vi "sub vi - Read Analog All v8.vi"(0 "Task0":dbl, 5 "Task1":dbl, 7 "Task2":dbl, 9 "Samples":dbl) -> (2 "Analog loop time":dbl, 3 "array GRAPH":dynamicdata[](array[waveform]), 4 "LAB01":T2, 6 "LAB02":T3, 8 "LAB03":T4, 10 "LAB04":T5, 13 "deg C":dbl, 14 "array ERROR":errorcluster[](array[cluster]), 15 "LAB05":T6)   [LabVIEW 2013]
uses:
  <vilib>/addons/Electrical Power/Basic/Measurement/Power (1 Channel).vi
  <vilib>/addons/Electrical Power/Basic/Measurement/RMS (N Channels).vi
  <vilib>/addons/Electrical Power/Basic/Measurement/RMS (1 Channel).vi
  <vilib>/addons/Electrical Power/Basic/NI_EP_Basic.lvlib
panel:
  in  "Tab Control":T1(tab)
  out "LAB01-2 (PF)":dbl
  out "LAB01-1 (PF)":dbl
  out "LAB01-2 (V)":dbl
  out "LAB01-2 (A)":dbl
  out "LAB01-1 (V)":dbl
  out "LAB01-1 (A)":dbl
  out "LAB01-2 (GRAPH)":dynamicdata(graph)
  out "LAB01-1 (GRAPH)":dynamicdata(graph)
  out "LAB02-2 (PF)":dbl
  out "LAB02-1 (PF)":dbl
  out "LAB02-2 (V)":dbl
  out "LAB02-2 (A)":dbl
  out "LAB02-1 (V)":dbl
  out "LAB02-1 (A)":dbl
  out "LAB02-2 (GRAPH)":dynamicdata(graph)
  out "LAB02-1 (GRAPH)":dynamicdata(graph)
  out "LAB03-2 (PF)":dbl
  out "LAB03-1 (PF)":dbl
  out "LAB03-2 (V)":dbl
  out "LAB03-2 (A)":dbl
  out "LAB03-1 (V)":dbl
  out "LAB03-1 (A)":dbl
  out "LAB03-2 (GRAPH)":dynamicdata(graph)
  out "LAB03-1 (GRAPH)":dynamicdata(graph)
  out "LAB04-2 (PF)":dbl
  out "LAB04-1 (PF)":dbl
  out "LAB04-2 (V)":dbl
  out "LAB04-2 (A)":dbl
  out "LAB04-1 (V)":dbl
  out "LAB04-1 (A)":dbl
  out "LAB04-1 (GRAPH)":dynamicdata(graph)
  out "LAB04-2 (GRAPH)":dynamicdata(graph)
  out "LAB05-2 (PF)":dbl
  out "LAB05-1 (PF)":dbl
  out "LAB05-2 (V)":dbl
  out "LAB05-2 (A)":dbl
  out "LAB05-1 (V)":dbl
  out "LAB05-1 (A)":dbl
  out "LAB05-1 (GRAPH)":dynamicdata(graph)
  out "LAB05-2 (GRAPH)":dynamicdata(graph)
  out "A1 error":errorcluster
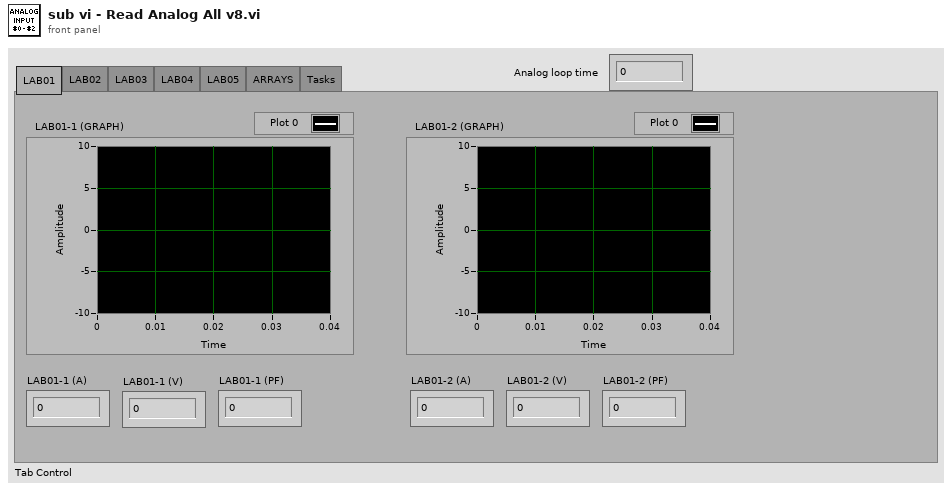
[diagram p1: front panel]
types:
  T1 = enum32{"LAB01", "LAB02", "LAB03", "LAB04", "LAB05", "ARRAYS", "Tasks"}
  T2 = cluster{"LAB01-1 (A)":dbl, "LAB01-1 (V)":dbl, "LAB01-1 (PF)":dbl, "LAB01-2 (A)":dbl, "LAB01-2 (V)":dbl, "LAB01-2 (PF)":dbl}
  T3 = cluster{"LAB02-1 (A)":dbl, "LAB02-1 (V)":dbl, "LAB02-1 (PF)":dbl, "LAB02-2 (A)":dbl, "LAB02-2 (V)":dbl, "LAB02-2 (PF)":dbl}
  T4 = cluster{"LAB03-1 (A)":dbl, "LAB03-1 (V)":dbl, "LAB03-1 (PF)":dbl, "LAB03-2 (A)":dbl, "LAB03-2 (V)":dbl, "LAB03-2 (PF)":dbl}
  T5 = cluster{"LAB04-1 (A)":dbl, "LAB04-1 (V)":dbl, "LAB04-1 (PF)":dbl, "LAB04-2 (A)":dbl, "LAB04-2 (V)":dbl, "LAB04-2 (PF)":dbl}
  T6 = cluster{"LAB05-1 (A)":dbl, "LAB05-1 (V)":dbl, "LAB05-1 (PF)":dbl, "LAB05-2 (A)":dbl, "LAB05-2 (V)":dbl, "LAB05-2 (PF)":dbl}
  T7 = typedef "NI_EP_Basic.lvlib/basic_Power Value.ctl" = cluster{"active power [W]":dbl, "apparent power [VA]":dbl, "reactive power [VAR]":dbl, "power factor":dbl}
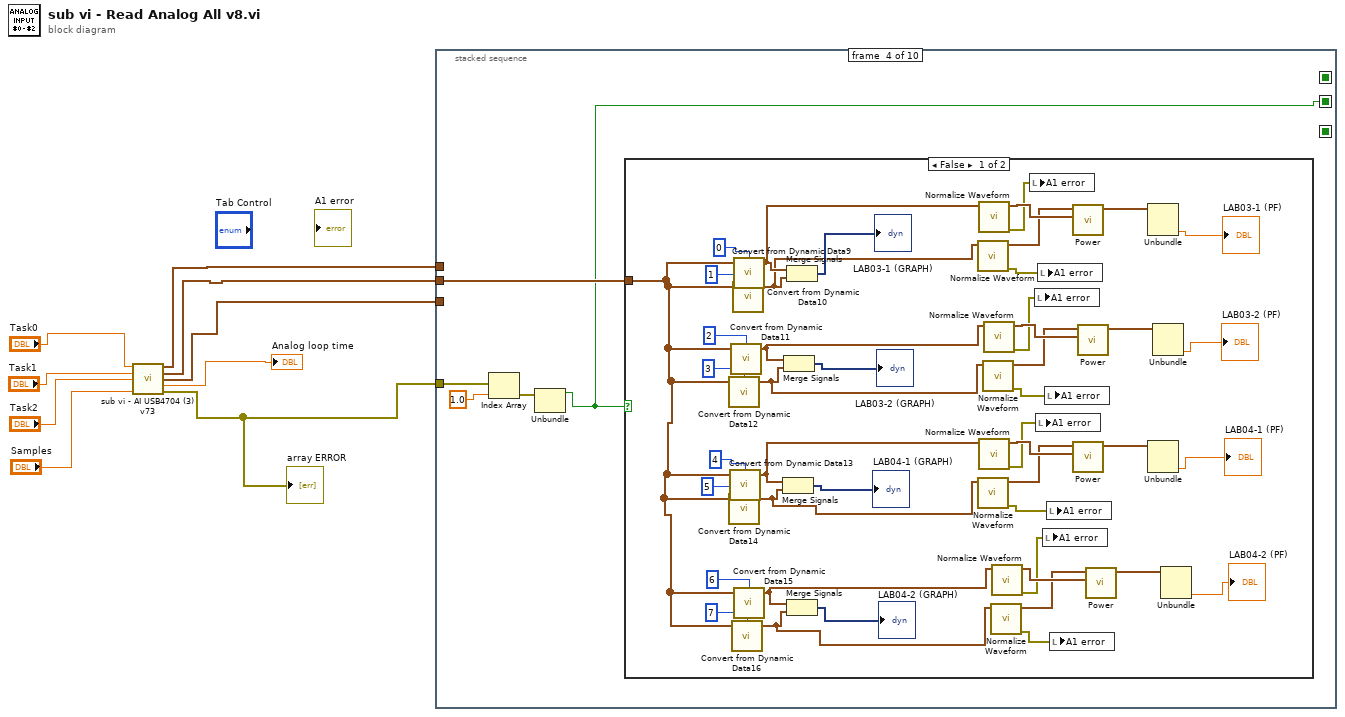
[diagram p0: block diagram]
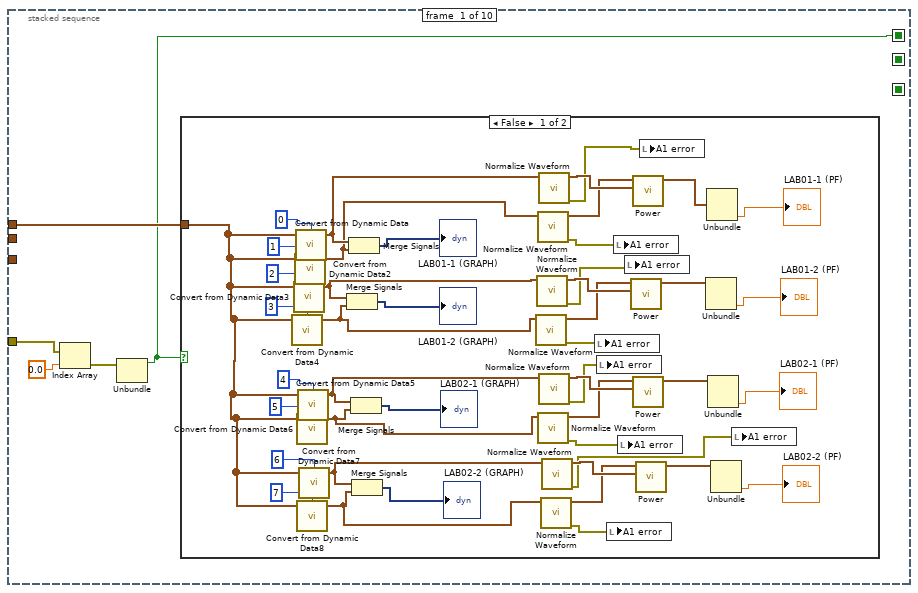
[diagram p2: hidden frame]
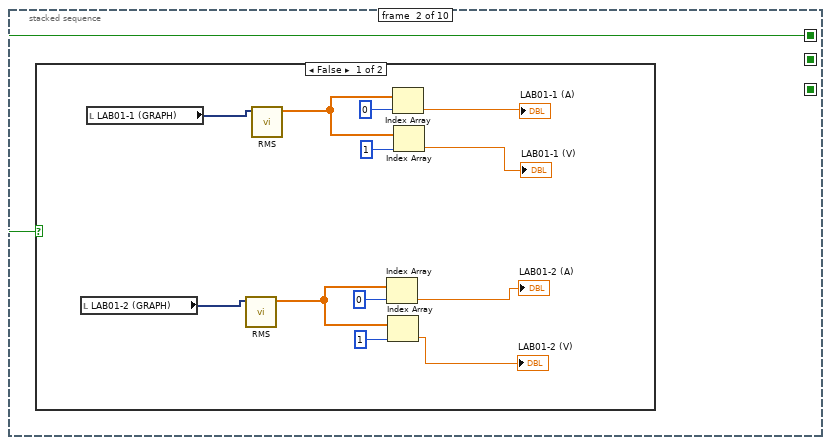
[diagram p4: hidden frame]
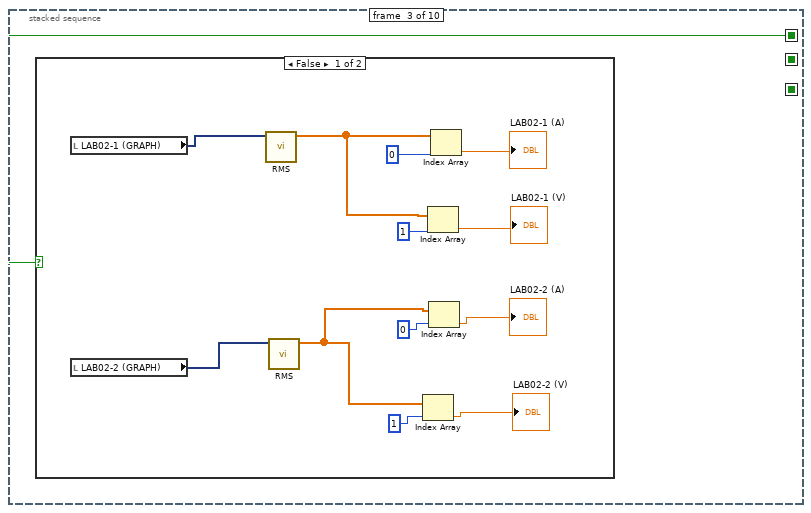
[diagram p6: hidden frame]
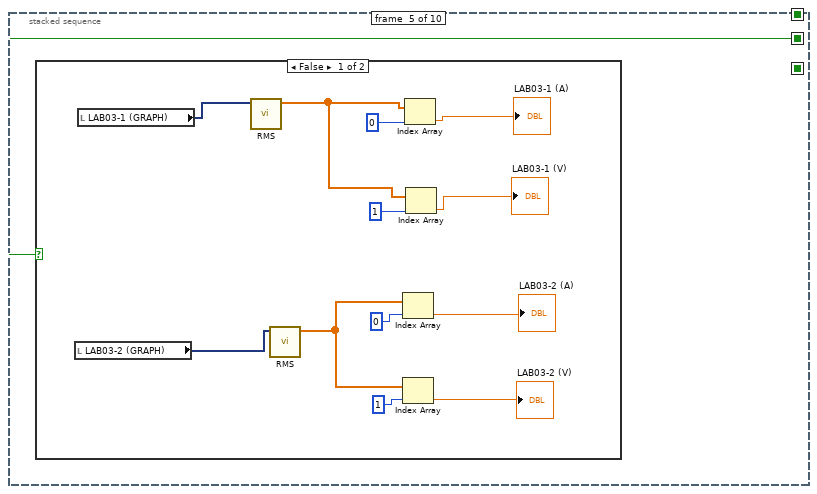
[diagram p9: hidden frame]
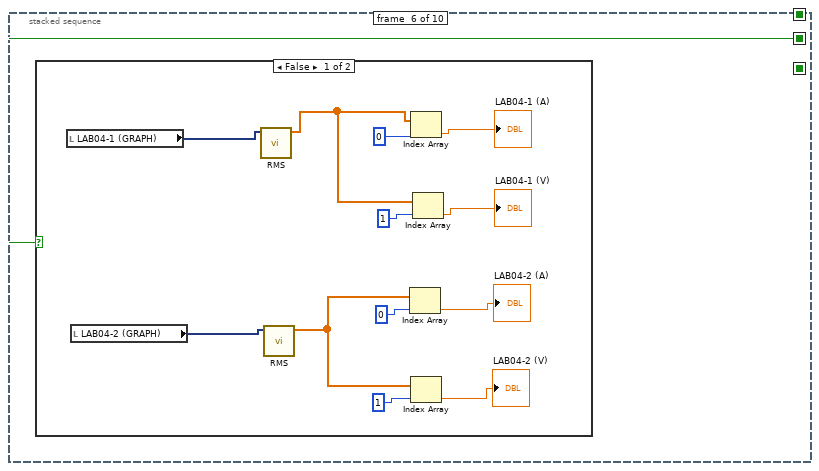
[diagram p11: hidden frame]
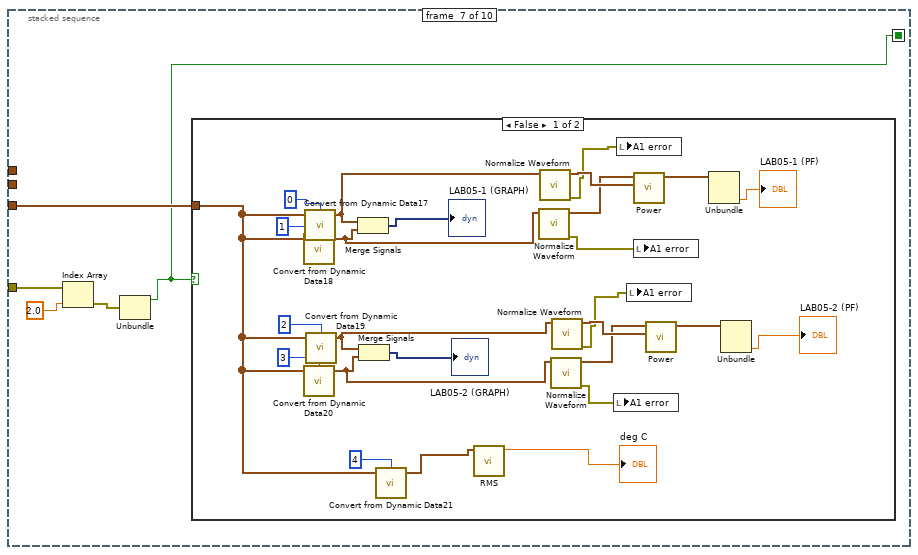
[diagram p13: hidden frame]
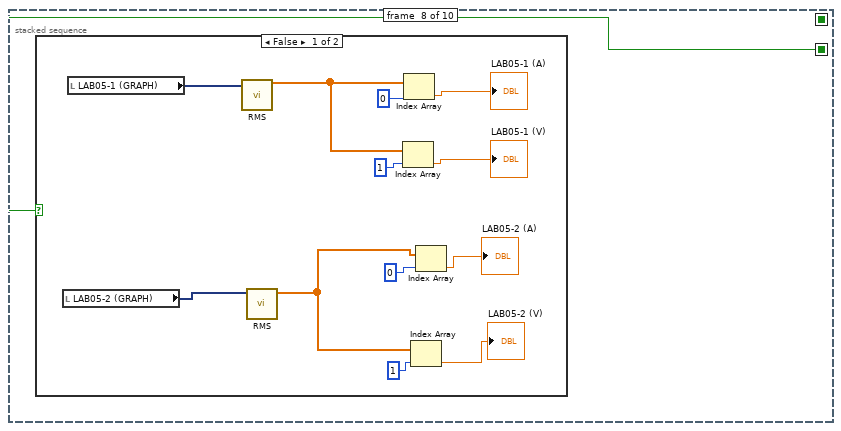
[diagram p15: hidden frame]
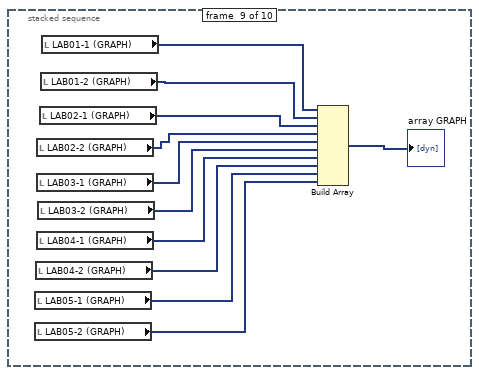
[diagram p17: hidden frame]
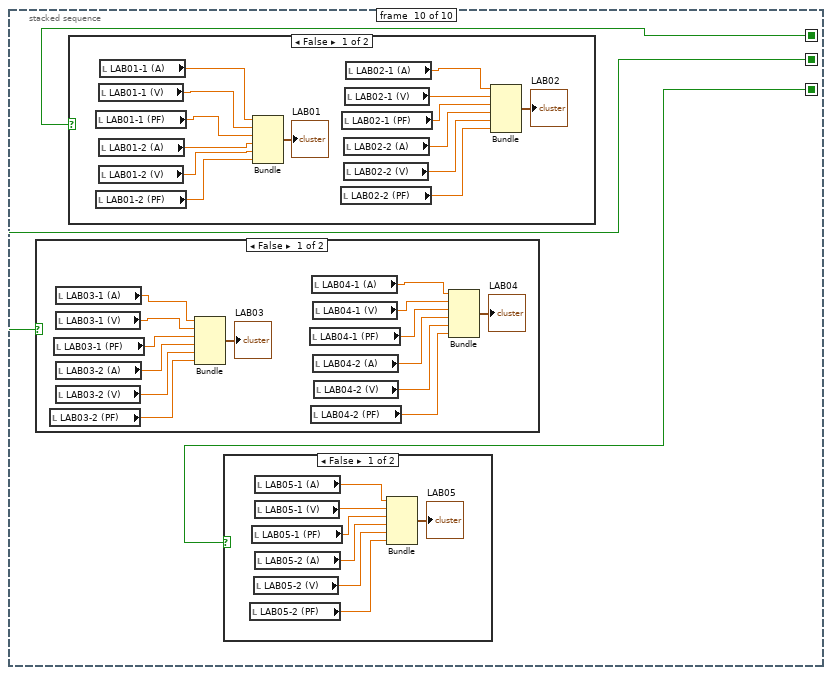
[diagram p18: hidden frame]
diagram:
  n1 = call "sub vi - AI USB4704 (3) v73.vi"("Task0"="Task0", "Task1"="Task1", "Task2"="Task2", "SAMPLES"="Samples") -> ("data 0"=w9:waveform(dbl)[], "data 1"=w8:waveform(dbl)[], "data 2"=w7:waveform(dbl)[], "loop time"=→"Analog loop time":dbl, "error array"=w5:errorcluster[])  [unwired: 7 in]
  "array ERROR" <- w5
  n2 = stacked-sequence {
    seq-local: [w10 _ _ _ _ _ _ _ _ _] -> [_ w60 w73 _ _ _ _ _ _ w219]
    seq-local: [_ _ _ w86 _ _ _ _ _ _] -> [_ _ _ _ w136 w149 _ _ _ w218]
    seq-local: [_ _ _ _ _ _ w162 _ _ _] -> [_ _ _ _ _ _ _ w193 _ w217]
    tunnel: w9 -> [w14 _ _ _ _ _ _ _ _ _]
    tunnel: w8 -> [_ _ _ w90 _ _ _ _ _ _]
    tunnel: w7 -> [_ _ _ _ _ _ w166 _ _ _]
    tunnel: w5 -> [w13 _ _ w89 _ _ w165 _ _ _]
    frame #0 {
      n3 = Index Array(array=w13, index=0.0) -> (element=w11:errorcluster)
      n4 = Unbundle(w11) -> ("status"=w10:bool)  [unwired: 2 out]
      n5 = case shown="False" w10 {
        tunnel: w14 -> [w49 _]
        frame False {
          n6 = call "Convert from Dynamic Data4"("Dynamic Data Type"=w49, "Channel"=3) -> ("Waveform"=w35:waveform(dbl))  [unwired: 2 in]
          n7 = call "Convert from Dynamic Data3"("Dynamic Data Type"=w49, "Channel"=2) -> ("Waveform"=w36:waveform(dbl))  [unwired: 2 in]
          n8 = call "Convert from Dynamic Data2"("Dynamic Data Type"=w49, "Channel"=1) -> ("Waveform"=w45:waveform(dbl))  [unwired: 2 in]
          n9 = call "Convert from Dynamic Data"("Dynamic Data Type"=w49, "Channel"=0) -> ("Waveform"=w46:waveform(dbl))  [unwired: 2 in]
          n10 = call "Convert from Dynamic Data6"("Dynamic Data Type"=w49, "Channel"=5) -> ("Waveform"=w30:waveform(dbl))  [unwired: 2 in]
          n11 = call "Convert from Dynamic Data8"("Dynamic Data Type"=w49, "Channel"=7) -> ("Waveform"=w24:waveform(dbl))  [unwired: 2 in]
          n12 = call "Convert from Dynamic Data5"("Dynamic Data Type"=w49, "Channel"=4) -> ("Waveform"=w31:waveform(dbl))  [unwired: 2 in]
          n13 = call "Convert from Dynamic Data7"("Dynamic Data Type"=w49, "Channel"=6) -> ("Waveform"=w25:waveform(dbl))  [unwired: 2 in]
          n14 = Merge Signals(w36, w35) -> (→"LAB01-2 (GRAPH)":dynamicdata)
          n15 = Merge Signals(w46, w45) -> (→"LAB01-1 (GRAPH)":dynamicdata)
          n16 = Merge Signals(w31, w30) -> (→"LAB02-1 (GRAPH)":dynamicdata)
          n17 = Merge Signals(w25, w24) -> (→"LAB02-2 (GRAPH)":dynamicdata)
          n18 = call <vilib>:"Normalize Waveform.vi"("waveform in"=w35) -> ("error out"=w19:errorcluster, "normalized waveform"=w39:waveform(dbl))  [unwired: 7 in, 2 out]
          n19 = call <vilib>:"Normalize Waveform.vi"("waveform in"=w36) -> ("error out"=w20:errorcluster, "normalized waveform"=w40:waveform(dbl))  [unwired: 7 in, 2 out]
          n20 = call <vilib>:"Normalize Waveform.vi"("waveform in"=w45) -> ("error out"=w21:errorcluster, "normalized waveform"=w43:waveform(dbl))  [unwired: 7 in, 2 out]
          n21 = call <vilib>:"Normalize Waveform.vi"("waveform in"=w30) -> ("error out"=w17:errorcluster, "normalized waveform"=w33:waveform(dbl))  [unwired: 7 in, 2 out]
          n22 = call <vilib>:"Normalize Waveform.vi"("waveform in"=w46) -> ("error out"=w22:errorcluster, "normalized waveform"=w44:waveform(dbl))  [unwired: 7 in, 2 out]
          n23 = call <vilib>:"Normalize Waveform.vi"("waveform in"=w31) -> ("error out"=w18:errorcluster, "normalized waveform"=w34:waveform(dbl))  [unwired: 7 in, 2 out]
          n24 = call <vilib>:"Normalize Waveform.vi"("waveform in"=w24) -> ("error out"=w15:errorcluster, "normalized waveform"=w27:waveform(dbl))  [unwired: 7 in, 2 out]
          n25 = call <vilib>:"Normalize Waveform.vi"("waveform in"=w25) -> ("error out"=w16:errorcluster, "normalized waveform"=w28:waveform(dbl))  [unwired: 7 in, 2 out]
          n26 = local write "A1 error"(w19) -> ()
          n27 = local write "A1 error"(w18) -> ()
          n28 = local write "A1 error"(w15) -> ()
          n29 = local write "A1 error"(w21) -> ()
          n30 = local write "A1 error"(w17) -> ()
          n31 = local write "A1 error"(w20) -> ()
          n32 = call-poly <vilib>:"Power.vi"("current waveform"=w40, "voltage waveform"=w39) -> ("power value"=w38:T7)  [unwired: 8 in, 1 out]
          n33 = call-poly <vilib>:"Power.vi"("current waveform"=w44, "voltage waveform"=w43) -> ("power value"=w42:T7)  [unwired: 8 in, 1 out]
          n34 = call-poly <vilib>:"Power.vi"("current waveform"=w34, "voltage waveform"=w33) -> ("power value"=w32:T7)  [unwired: 8 in, 1 out]
          n35 = call-poly <vilib>:"Power.vi"("current waveform"=w28, "voltage waveform"=w27) -> ("power value"=w26:T7)  [unwired: 8 in, 1 out]
          n36 = local write "A1 error"(w22) -> ()
          n37 = Unbundle(w38) -> ("power factor"=→"LAB01-2 (PF)":dbl)  [unwired: 3 out]
          n38 = Unbundle(w42) -> ("power factor"=→"LAB01-1 (PF)":dbl)  [unwired: 3 out]
          n39 = Unbundle(w32) -> ("power factor"=→"LAB02-1 (PF)":dbl)  [unwired: 3 out]
          n40 = Unbundle(w26) -> ("power factor"=→"LAB02-2 (PF)":dbl)  [unwired: 3 out]
          n41 = local write "A1 error"(w16) -> ()
        }
        frame True {
        }
      }
    }
    frame #1 {
      n42 = case shown="False" w60 {
        frame False {
          n43 = local read "LAB01-2 (GRAPH)"() -> (w69:dynamicdata)
          n44 = local read "LAB01-1 (GRAPH)"() -> (w63:dynamicdata)
          n45 = call-poly <vilib>:"RMS.vi"("waveforms"=w69) -> ("RMS values"=w68:dbl[])  [unwired: 9 in, 1 out]
          n46 = call-poly <vilib>:"RMS.vi"("waveforms"=w63) -> ("RMS values"=w72:dbl[])  [unwired: 9 in, 1 out]
          n47 = Index Array(array=w68, index=0) -> (element=→"LAB01-2 (A)":dbl)
          n48 = Index Array(array=w68, index=1) -> (element=→"LAB01-2 (V)":dbl)
          n49 = Index Array(array=w72, index=0) -> (element=→"LAB01-1 (A)":dbl)
          n50 = Index Array(array=w72, index=1) -> (element=→"LAB01-1 (V)":dbl)
        }
        frame True {
        }
      }
    }
    frame #2 {
      n51 = case shown="False" w73 {
        frame False {
          n52 = local read "LAB02-1 (GRAPH)"() -> (w81:dynamicdata)
          n53 = local read "LAB02-2 (GRAPH)"() -> (w77:dynamicdata)
          n54 = call-poly <vilib>:"RMS.vi"("waveforms"=w81) -> ("RMS values"=w80:dbl[])  [unwired: 9 in, 1 out]
          n55 = call-poly <vilib>:"RMS.vi"("waveforms"=w77) -> ("RMS values"=w76:dbl[])  [unwired: 9 in, 1 out]
          n56 = Index Array(array=w76, index=1) -> (element=→"LAB02-2 (V)":dbl)
          n57 = Index Array(array=w80, index=1) -> (element=→"LAB02-1 (V)":dbl)
          n58 = Index Array(array=w76, index=0) -> (element=→"LAB02-2 (A)":dbl)
          n59 = Index Array(array=w80, index=0) -> (element=→"LAB02-1 (A)":dbl)
        }
        frame True {
        }
      }
    }
    frame #3 {
      n60 = Index Array(array=w89, index=1.0) -> (element=w87:errorcluster)
      n61 = Unbundle(w87) -> ("status"=w86:bool)  [unwired: 2 out]
      n62 = case shown="False" w86 {
        tunnel: w90 -> [w123 _]
        frame False {
          n63 = call "Convert from Dynamic Data12"("Dynamic Data Type"=w123, "Channel"=3) -> ("Waveform"=w112:waveform(dbl))  [unwired: 2 in]
          n64 = call "Convert from Dynamic Data14"("Dynamic Data Type"=w123, "Channel"=5) -> ("Waveform"=w106:waveform(dbl))  [unwired: 2 in]
          n65 = call "Convert from Dynamic Data13"("Dynamic Data Type"=w123, "Channel"=4) -> ("Waveform"=w107:waveform(dbl))  [unwired: 2 in]
          n66 = call "Convert from Dynamic Data11"("Dynamic Data Type"=w123, "Channel"=2) -> ("Waveform"=w113:waveform(dbl))  [unwired: 2 in]
          n67 = call "Convert from Dynamic Data16"("Dynamic Data Type"=w123, "Channel"=7) -> ("Waveform"=w100:waveform(dbl))  [unwired: 2 in]
          n68 = call "Convert from Dynamic Data10"("Dynamic Data Type"=w123, "Channel"=1) -> ("Waveform"=w118:waveform(dbl))  [unwired: 2 in]
          n69 = call "Convert from Dynamic Data9"("Dynamic Data Type"=w123, "Channel"=0) -> ("Waveform"=w119:waveform(dbl))  [unwired: 2 in]
          n70 = call "Convert from Dynamic Data15"("Dynamic Data Type"=w123, "Channel"=6) -> ("Waveform"=w101:waveform(dbl))  [unwired: 2 in]
          n71 = Merge Signals(w107, w106) -> (→"LAB04-1 (GRAPH)":dynamicdata)
          n72 = Merge Signals(w113, w112) -> (→"LAB03-2 (GRAPH)":dynamicdata)
          n73 = Merge Signals(w119, w118) -> (→"LAB03-1 (GRAPH)":dynamicdata)
          n74 = Merge Signals(w101, w100) -> (→"LAB04-2 (GRAPH)":dynamicdata)
          n75 = call <vilib>:"Normalize Waveform.vi"("waveform in"=w118) -> ("error out"=w97:errorcluster, "normalized waveform"=w121:waveform(dbl))  [unwired: 7 in, 2 out]
          n76 = call <vilib>:"Normalize Waveform.vi"("waveform in"=w106) -> ("error out"=w93:errorcluster, "normalized waveform"=w109:waveform(dbl))  [unwired: 7 in, 2 out]
          n77 = call <vilib>:"Normalize Waveform.vi"("waveform in"=w119) -> ("error out"=w98:errorcluster, "normalized waveform"=w122:waveform(dbl))  [unwired: 7 in, 2 out]
          n78 = call <vilib>:"Normalize Waveform.vi"("waveform in"=w107) -> ("error out"=w94:errorcluster, "normalized waveform"=w110:waveform(dbl))  [unwired: 7 in, 2 out]
          n79 = call <vilib>:"Normalize Waveform.vi"("waveform in"=w112) -> ("error out"=w95:errorcluster, "normalized waveform"=w115:waveform(dbl))  [unwired: 7 in, 2 out]
          n80 = call <vilib>:"Normalize Waveform.vi"("waveform in"=w113) -> ("error out"=w96:errorcluster, "normalized waveform"=w116:waveform(dbl))  [unwired: 7 in, 2 out]
          n81 = call <vilib>:"Normalize Waveform.vi"("waveform in"=w100) -> ("error out"=w91:errorcluster, "normalized waveform"=w103:waveform(dbl))  [unwired: 7 in, 2 out]
          n82 = call <vilib>:"Normalize Waveform.vi"("waveform in"=w101) -> ("error out"=w92:errorcluster, "normalized waveform"=w104:waveform(dbl))  [unwired: 7 in, 2 out]
          n83 = local write "A1 error"(w98) -> ()
          n84 = local write "A1 error"(w96) -> ()
          n85 = local write "A1 error"(w94) -> ()
          n86 = local write "A1 error"(w97) -> ()
          n87 = local write "A1 error"(w92) -> ()
          n88 = local write "A1 error"(w95) -> ()
          n89 = local write "A1 error"(w93) -> ()
          n90 = local write "A1 error"(w91) -> ()
          n91 = call-poly <vilib>:"Power.vi"("current waveform"=w122, "voltage waveform"=w121) -> ("power value"=w120:T7)  [unwired: 8 in, 1 out]
          n92 = call-poly <vilib>:"Power.vi"("current waveform"=w110, "voltage waveform"=w109) -> ("power value"=w108:T7)  [unwired: 8 in, 1 out]
          n93 = call-poly <vilib>:"Power.vi"("current waveform"=w116, "voltage waveform"=w115) -> ("power value"=w114:T7)  [unwired: 8 in, 1 out]
          n94 = call-poly <vilib>:"Power.vi"("current waveform"=w104, "voltage waveform"=w103) -> ("power value"=w102:T7)  [unwired: 8 in, 1 out]
          n95 = Unbundle(w120) -> ("power factor"=→"LAB03-1 (PF)":dbl)  [unwired: 3 out]
          n96 = Unbundle(w108) -> ("power factor"=→"LAB04-1 (PF)":dbl)  [unwired: 3 out]
          n97 = Unbundle(w114) -> ("power factor"=→"LAB03-2 (PF)":dbl)  [unwired: 3 out]
          n98 = Unbundle(w102) -> ("power factor"=→"LAB04-2 (PF)":dbl)  [unwired: 3 out]
        }
        frame True {
        }
      }
    }
    frame #4 {
      n99 = case shown="False" w136 {
        frame False {
          n100 = local read "LAB03-2 (GRAPH)"() -> (w143:dynamicdata)
          n101 = local read "LAB03-1 (GRAPH)"() -> (w144:dynamicdata)
          n102 = call-poly <vilib>:"RMS.vi"("waveforms"=w144) -> ("RMS values"=w142:dbl[])  [unwired: 9 in, 1 out]
          n103 = call-poly <vilib>:"RMS.vi"("waveforms"=w143) -> ("RMS values"=w139:dbl[])  [unwired: 9 in, 1 out]
          n104 = Index Array(array=w139, index=0) -> (element=→"LAB03-2 (A)":dbl)
          n105 = Index Array(array=w139, index=1) -> (element=→"LAB03-2 (V)":dbl)
          n106 = Index Array(array=w142, index=0) -> (element=→"LAB03-1 (A)":dbl)
          n107 = Index Array(array=w142, index=1) -> (element=→"LAB03-1 (V)":dbl)
        }
        frame True {
        }
      }
    }
    frame #5 {
      n108 = case shown="False" w149 {
        frame False {
          n109 = local read "LAB04-1 (GRAPH)"() -> (w157:dynamicdata)
          n110 = local read "LAB04-2 (GRAPH)"() -> (w153:dynamicdata)
          n111 = call-poly <vilib>:"RMS.vi"("waveforms"=w157) -> ("RMS values"=w156:dbl[])  [unwired: 9 in, 1 out]
          n112 = call-poly <vilib>:"RMS.vi"("waveforms"=w153) -> ("RMS values"=w152:dbl[])  [unwired: 9 in, 1 out]
          n113 = Index Array(array=w152, index=0) -> (element=→"LAB04-2 (A)":dbl)
          n114 = Index Array(array=w156, index=0) -> (element=→"LAB04-1 (A)":dbl)
          n115 = Index Array(array=w152, index=1) -> (element=→"LAB04-2 (V)":dbl)
          n116 = Index Array(array=w156, index=1) -> (element=→"LAB04-1 (V)":dbl)
        }
        frame True {
        }
      }
    }
    frame #6 {
      n117 = Index Array(array=w165, index=2.0) -> (element=w163:errorcluster)
      n118 = Unbundle(w163) -> ("status"=w162:bool)  [unwired: 2 out]
      n119 = case shown="False" w162 {
        tunnel: w166 -> [w169 _]
        frame False {
          n120 = call "Convert from Dynamic Data18"("Dynamic Data Type"=w169, "Channel"=1) -> ("Waveform"=w182:waveform(dbl))  [unwired: 2 in]
          n121 = call "Convert from Dynamic Data20"("Dynamic Data Type"=w169, "Channel"=3) -> ("Waveform"=w176:waveform(dbl))  [unwired: 2 in]
          n122 = call "Convert from Dynamic Data17"("Dynamic Data Type"=w169, "Channel"=0) -> ("Waveform"=w183:waveform(dbl))  [unwired: 2 in]
          n123 = call "Convert from Dynamic Data19"("Dynamic Data Type"=w169, "Channel"=2) -> ("Waveform"=w177:waveform(dbl))  [unwired: 2 in]
          n124 = Merge Signals(w183, w182) -> (→"LAB05-1 (GRAPH)":dynamicdata)
          n125 = Merge Signals(w177, w176) -> (→"LAB05-2 (GRAPH)":dynamicdata)
          n126 = call "Convert from Dynamic Data21"("Dynamic Data Type"=w169, "Channel"=4) -> ("Waveform"=w168:waveform(dbl))  [unwired: 2 in]
          n127 = call-poly <vilib>:"RMS.vi"("waveform"=w168) -> ("RMS value"=→"deg C":dbl)  [unwired: 9 in, 1 out]
          n128 = call <vilib>:"Normalize Waveform.vi"("waveform in"=w182) -> ("error out"=w174:errorcluster, "normalized waveform"=w185:waveform(dbl))  [unwired: 7 in, 2 out]
          n129 = call <vilib>:"Normalize Waveform.vi"("waveform in"=w183) -> ("error out"=w173:errorcluster, "normalized waveform"=w186:waveform(dbl))  [unwired: 7 in, 2 out]
          n130 = call <vilib>:"Normalize Waveform.vi"("waveform in"=w176) -> ("error out"=w172:errorcluster, "normalized waveform"=w179:waveform(dbl))  [unwired: 7 in, 2 out]
          n131 = call <vilib>:"Normalize Waveform.vi"("waveform in"=w177) -> ("error out"=w171:errorcluster, "normalized waveform"=w180:waveform(dbl))  [unwired: 7 in, 2 out]
          n132 = local write "A1 error"(w172) -> ()
          n133 = local write "A1 error"(w173) -> ()
          n134 = local write "A1 error"(w171) -> ()
          n135 = call-poly <vilib>:"Power.vi"("current waveform"=w186, "voltage waveform"=w185) -> ("power value"=w184:T7)  [unwired: 8 in, 1 out]
          n136 = local write "A1 error"(w174) -> ()
          n137 = call-poly <vilib>:"Power.vi"("current waveform"=w180, "voltage waveform"=w179) -> ("power value"=w178:T7)  [unwired: 8 in, 1 out]
          n138 = Unbundle(w184) -> ("power factor"=→"LAB05-1 (PF)":dbl)  [unwired: 3 out]
          n139 = Unbundle(w178) -> ("power factor"=→"LAB05-2 (PF)":dbl)  [unwired: 3 out]
        }
        frame True {
        }
      }
    }
    frame #7 {
      n140 = case shown="False" w193 {
        frame False {
          n141 = local read "LAB05-2 (GRAPH)"() -> (w200:dynamicdata)
          n142 = local read "LAB05-1 (GRAPH)"() -> (w201:dynamicdata)
          n143 = call-poly <vilib>:"RMS.vi"("waveforms"=w201) -> ("RMS values"=w199:dbl[])  [unwired: 9 in, 1 out]
          n144 = call-poly <vilib>:"RMS.vi"("waveforms"=w200) -> ("RMS values"=w198:dbl[])  [unwired: 9 in, 1 out]
          n145 = Index Array(array=w199, index=1) -> (element=→"LAB05-1 (V)":dbl)
          n146 = Index Array(array=w199, index=0) -> (element=→"LAB05-1 (A)":dbl)
          n147 = Index Array(array=w198, index=1) -> (element=→"LAB05-2 (V)":dbl)
          n148 = Index Array(array=w198, index=0) -> (element=→"LAB05-2 (A)":dbl)
        }
        frame True {
        }
      }
    }
    frame #8 {
      n149 = local read "LAB05-1 (GRAPH)"() -> (w208:dynamicdata)
      n150 = local read "LAB05-2 (GRAPH)"() -> (w207:dynamicdata)
      n151 = local read "LAB04-2 (GRAPH)"() -> (w209:dynamicdata)
      n152 = local read "LAB02-2 (GRAPH)"() -> (w213:dynamicdata)
      n153 = local read "LAB03-1 (GRAPH)"() -> (w212:dynamicdata)
      n154 = local read "LAB04-1 (GRAPH)"() -> (w210:dynamicdata)
      n155 = local read "LAB03-2 (GRAPH)"() -> (w211:dynamicdata)
      n156 = local read "LAB02-1 (GRAPH)"() -> (w214:dynamicdata)
      n157 = local read "LAB01-2 (GRAPH)"() -> (w215:dynamicdata)
      n158 = local read "LAB01-1 (GRAPH)"() -> (w216:dynamicdata)
      n159 = Build Array(w216, w215, w214, w213, w212, w211, w210, w209, w208, w207) -> (→"array GRAPH":dynamicdata[])
    }
    frame #9 {
      n160 = case shown="False" w218 {
        frame False {
          n161 = local read "LAB03-2 (PF)"() -> (w235:dbl)
          n162 = local read "LAB03-1 (PF)"() -> (w238:dbl)
          n163 = local read "LAB03-1 (A)"() -> (w240:dbl)
          n164 = local read "LAB03-1 (V)"() -> (w239:dbl)
          n165 = local read "LAB03-2 (A)"() -> (w237:dbl)
          n166 = local read "LAB03-2 (V)"() -> (w236:dbl)
          n167 = Bundle("LAB03-1 (A)"=w240, "LAB03-1 (V)"=w239, "LAB03-1 (PF)"=w238, "LAB03-2 (A)"=w237, "LAB03-2 (V)"=w236, "LAB03-2 (PF)"=w235) -> (→"LAB03":T4)  [unwired: 1 in]
          n168 = local read "LAB04-1 (PF)"() -> (w232:dbl)
          n169 = local read "LAB04-2 (PF)"() -> (w229:dbl)
          n170 = local read "LAB04-1 (A)"() -> (w234:dbl)
          n171 = local read "LAB04-1 (V)"() -> (w233:dbl)
          n172 = local read "LAB04-2 (A)"() -> (w231:dbl)
          n173 = local read "LAB04-2 (V)"() -> (w230:dbl)
          n174 = Bundle("LAB04-1 (A)"=w234, "LAB04-1 (V)"=w233, "LAB04-1 (PF)"=w232, "LAB04-2 (A)"=w231, "LAB04-2 (V)"=w230, "LAB04-2 (PF)"=w229) -> (→"LAB04":T5)  [unwired: 1 in]
        }
        frame True {
        }
      }
      n175 = case shown="False" w219 {
        frame False {
          n176 = local read "LAB01-1 (PF)"() -> (w245:dbl)
          n177 = local read "LAB01-2 (PF)"() -> (w242:dbl)
          n178 = local read "LAB01-1 (V)"() -> (w246:dbl)
          n179 = local read "LAB01-2 (A)"() -> (w244:dbl)
          n180 = local read "LAB01-2 (V)"() -> (w243:dbl)
          n181 = local read "LAB01-1 (A)"() -> (w247:dbl)
          n182 = Bundle("LAB01-1 (A)"=w247, "LAB01-1 (V)"=w246, "LAB01-1 (PF)"=w245, "LAB01-2 (A)"=w244, "LAB01-2 (V)"=w243, "LAB01-2 (PF)"=w242) -> (→"LAB01":T2)  [unwired: 1 in]
          n183 = local read "LAB02-2 (PF)"() -> (w249:dbl)
          n184 = local read "LAB02-1 (PF)"() -> (w252:dbl)
          n185 = local read "LAB02-2 (A)"() -> (w251:dbl)
          n186 = local read "LAB02-2 (V)"() -> (w250:dbl)
          n187 = local read "LAB02-1 (V)"() -> (w253:dbl)
          n188 = local read "LAB02-1 (A)"() -> (w254:dbl)
          n189 = Bundle("LAB02-1 (A)"=w254, "LAB02-1 (V)"=w253, "LAB02-1 (PF)"=w252, "LAB02-2 (A)"=w251, "LAB02-2 (V)"=w250, "LAB02-2 (PF)"=w249) -> (→"LAB02":T3)  [unwired: 1 in]
        }
        frame True {
        }
      }
      n190 = case shown="False" w217 {
        frame False {
          n191 = local read "LAB05-2 (PF)"() -> (w221:dbl)
          n192 = local read "LAB05-1 (PF)"() -> (w224:dbl)
          n193 = local read "LAB05-2 (V)"() -> (w222:dbl)
          n194 = local read "LAB05-1 (A)"() -> (w226:dbl)
          n195 = local read "LAB05-1 (V)"() -> (w225:dbl)
          n196 = local read "LAB05-2 (A)"() -> (w223:dbl)
          n197 = Bundle("LAB05-1 (A)"=w226, "LAB05-1 (V)"=w225, "LAB05-1 (PF)"=w224, "LAB05-2 (A)"=w223, "LAB05-2 (V)"=w222, "LAB05-2 (PF)"=w221) -> (→"LAB05":T6)  [unwired: 1 in]
        }
        frame True {
        }
      }
    }
  }
